vi "GetAllChildrenRecursive.vi"(0 "reference":refnum<class "AbstractNode.lvclass">, 5 "error in (no error)":errorcluster) -> (14 "reference out":refnum<class "AbstractNode.lvclass">, 15 "children":refnum<class "AbstractNode.lvclass">[](array[class]), 19 "error out":errorcluster)   [LabVIEW 2020, in "AbstractNode.lvclass"]
doc: "GetAllChildrenRecursive"
uses:
  <resource>/Framework/Providers/Open_GDS/UML/AbstractNode_class/AbstractNode.lvclass
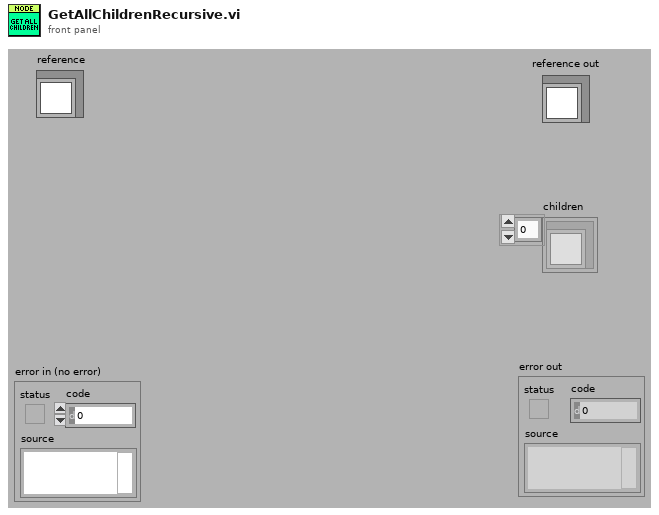
[diagram p1: front panel]
types:
  T1 = typedef "AbstractNode.lvclass/ObjectAttributes.ctl" = cluster{"parent":refnum<class "AbstractNode.lvclass">, "children":refnum<class "AbstractNode.lvclass">[], "Hidden":bool}
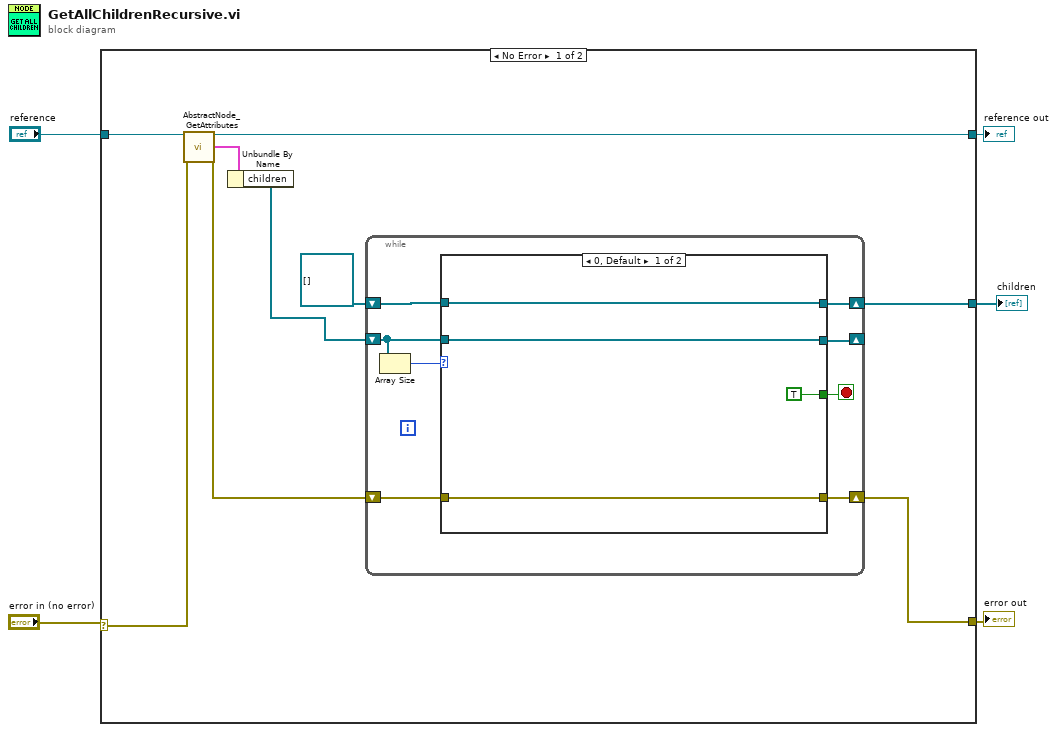
[diagram p0: block diagram]
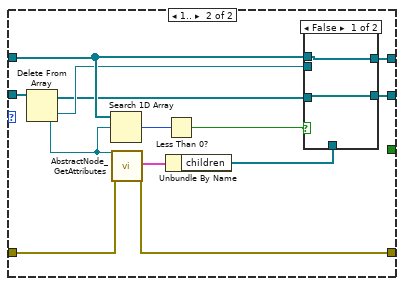
[diagram p2: hidden frame]
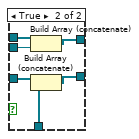
[diagram p3: hidden frame]
diagram:
  n1 = case shown="No Error" "error in (no error)" {
    selector: "error in (no error)" -> [w12 w47]
    tunnel: "reference" -> [w14 w48]
    tunnel: [w10 w47] -> w4
    tunnel: [w13 w48] -> w3
    tunnel: [w8 _] -> w1
    frame No Error {
      n2 = call <resource>:"AbstractNode_GetAttributes.vi"("reference in"=w14, "error in (no error)"=w12) -> ("reference out"=w13:refnum<class "AbstractNode.lvclass">, "Data"=w6:T1, "error out"=w11:errorcluster)  [unwired: 1 in, 14 out]
      n3 = Unbundle By Name(w6) -> ("children"=w9:refnum<class "AbstractNode.lvclass">[])
      n4 = while {
        shift-right: [w22] -> w8
        shift-left: refnum<class "AbstractNode.lvclass">[] [] -> [w19]
        shift-right: [w20] -> w10
        shift-left: w11 -> [w21]
        shift-right: [w16] -> _
        shift-left: w9 -> [w15]
        stop <- w17 stop-if-true
        n5 = Array Size(array=w15) -> (size(s)=w18:i32)
        n6 = case shown="0, Default" w18 {
          tunnel: [w24 w38] -> w22
          tunnel: w21 -> [w25 w37]
          tunnel: [w25 w36] -> w20
          tunnel: w19 -> [w24 w34]
          tunnel: [TRUE _] -> w17
          tunnel: [w23 w29] -> w16
          tunnel: w15 -> [w23 w35]
          frame 0, Default {
          }
          frame 1.. {
            n7 = Delete From Array(array=w35) -> (deleted portion=w32:refnum<class "AbstractNode.lvclass">, array with subset deleted=w30:refnum<class "AbstractNode.lvclass">[])  [unwired: 2 in]
            n8 = Search 1D Array(1D array=w34, element=w32) -> (index of element=w33:i32)  [unwired: 1 in]
            n9 = call <resource>:"AbstractNode_GetAttributes.vi"("reference in"=w32, "error in (no error)"=w37) -> ("Data"=w27:T1, "error out"=w36:errorcluster)  [unwired: 1 in, 15 out]
            n10 = Less Than 0?(x=w33) -> (x < 0?=w31:bool)
            n11 = Unbundle By Name(w27) -> ("children"=w28:refnum<class "AbstractNode.lvclass">[])
            n12 = case shown="False" w31 {
              tunnel: [w40 w43] -> w38
              tunnel: w34 -> [w40 w46]
              tunnel: w32 -> [_ w45]
              tunnel: w30 -> [w39 w44]
              tunnel: [w39 w42] -> w29
              tunnel: w28 -> [_ w41]
              frame False {
              }
              frame True {
                n13 = Build Array (concatenate)(w46, w45) -> (w43:refnum<class "AbstractNode.lvclass">[])
                n14 = Build Array (concatenate)(w44, w41) -> (w42:refnum<class "AbstractNode.lvclass">[])
              }
            }
          }
        }
      }
    }
    frame Error {
    }
  }
  "reference out" <- w3
  "error out" <- w4
  "children" <- w1
